vi "State_Machine.vi"(8 "error in (no error)":errorcluster caption="entrée d'erreur (pas d'erreur)", 11 "Get_Voltage en entrée":refnum<class "Zigbee_White_List.lvclass">) -> (0 "error out":errorcluster caption="sortie d'erreur", 2 "Json_String":string, 3 "Get_Voltage en sortie":refnum<class "Zigbee_White_List.lvclass">)   [LabVIEW 2020, in "Library Test.lvlib" / "Zigbee_White_List.lvclass"]
uses:
  Zigbee_White_List.lvclass
  C:/Users/ngarcin/OneDrive - Altyor/Standard TB/Suite TB45/Class/Test/Zigbee_Send_Command_UART/Zigbee_Send_Command_UART.lvclass
  Commun VI/TypeDef/Variable Printable.ctl
  Zigbee_Send_Command_UART/Zigbee_Send_Command_UART.lvclass
  Commun VI/Library Commun.lvlib
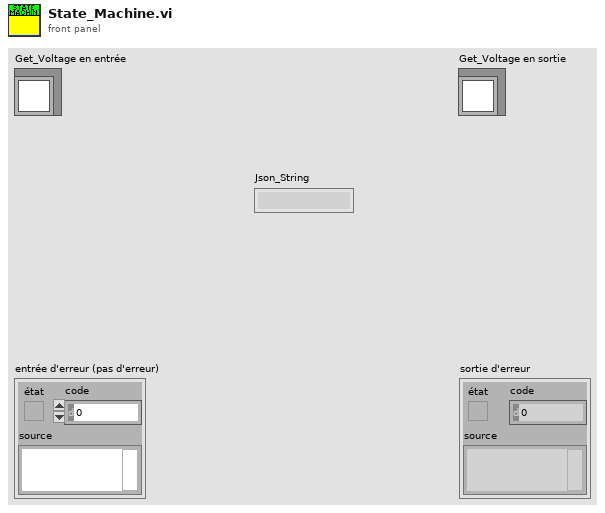
[diagram p1: front panel]
types:
  T1 = typedef "Variable Printable.ctl" = string
  T2 = enum16{"Get Variable", "Get All Variables", "Set Variable", "Delete Variable", "Delete All Variable"}
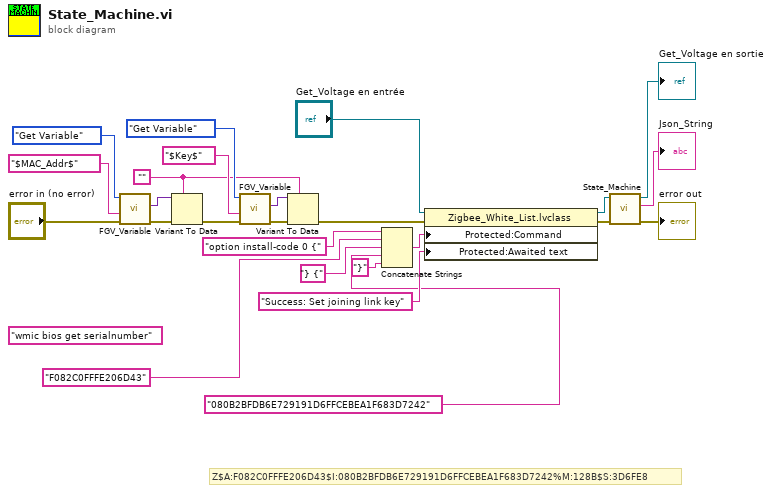
[diagram p0: block diagram]
diagram:
  w6 = ""
  (unwired) "wmic bios get serialnumber" ("command line")
  # "Z$A:F082C0FFFE206D43$I:080B2BFDB6E729191D6FFCEBEA1F683D7242%M:128B$S:3D6FE8"
  n1 = call "FGV_Variable.vi"("error in (no error)"="error in (no error)", "Variable"=T1 "$MAC_Addr$" ("Variable Printable"), "Function"=T2."Get Variable") -> ("error out"=w13:errorcluster, "Data Out"=w10:variant)  [unwired: 6 in, 1 out]
  n2 = Variant To Data(error in=w13, type=w6, Variant=w10) -> (error out=w12:errorcluster)  [unwired: 1 out]
  n3 = call "FGV_Variable.vi"("error in (no error)"=w12, "Variable"=T1 "$Key$" ("Variable Printable"), "Function"=T2."Get Variable") -> ("error out"=w9:errorcluster, "Data Out"=w8:variant)  [unwired: 6 in, 1 out]
  n4 = Variant To Data(error in=w9, type=w6, Variant=w8) -> (error out=w4:errorcluster)  [unwired: 1 out]
  n5 = Concatenate Strings("option install-code 0 {" ("Command"), "F082C0FFFE206D43", "} {" ("chaîne"), "080B2BFDB6E729191D6FFCEBEA1F683D7242", "}" ("chaîne")) -> (w19:string)
  n6 = property class="Zigbee_White_List.lvclass"(reference="Get_Voltage en entrée", error in=w4, "Protected:Command"=w19, "Protected:Awaited text"="Success: Set joining link key" ("Awaited text")) -> (reference out=w22:refnum<class "Zigbee_White_List.lvclass">, error out=w21:errorcluster)
  n7 = call-parent "State_Machine.vi"("error in (no error)"=w21, "Send_Frame en entrée"=w22) -> ("error out"=→"error out":errorcluster, "Json_String"=→"Json_String":string, "Send_Frame en sortie"=→"Get_Voltage en sortie":refnum<class "Zigbee_White_List.lvclass">)  [unwired: 7 in]
